vi "Is Last.vi"(8 "error in (no error)":errorcluster, 11 "Vector in":refnum<class "Vector Parent.lvclass">) -> (0 "error out":errorcluster, 2 "Last?":bool, 3 "Vector out":refnum<class "Vector Parent.lvclass">)   [LabVIEW 2019, in "Vector Parent.lvclass"]
uses:
  Vector Parent.lvclass
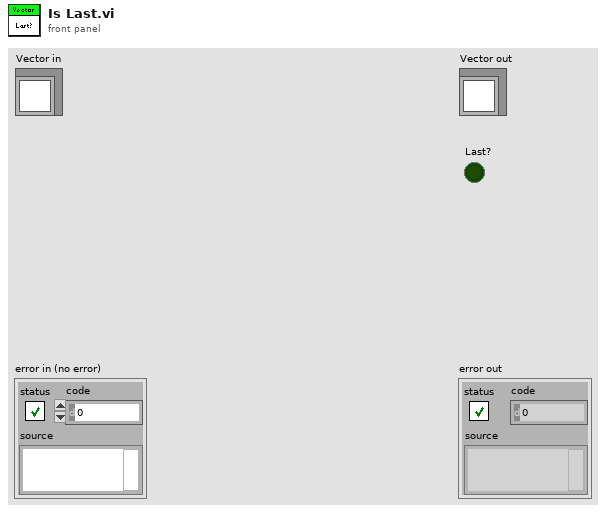
[diagram p1: front panel]
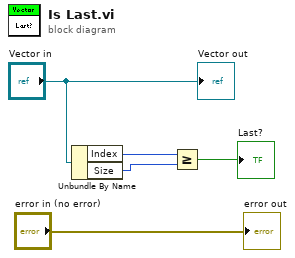
[diagram p0: block diagram]
diagram:
  n1 = Unbundle By Name("Vector in") -> ("Index"=w3:i32, "Size"=w4:u32)
  n2 = Greater Or Equal?(x=w3, y=w4) -> (x >= y?=→"Last?":bool)
  "error out" <- "error in (no error)"
  "Vector out" <- "Vector in"
